vi "PassObserverTactic.vi"(1 "Game in":refnum<class "Game.lvclass">, 8 "error in (no error)":errorcluster, 9 "first call":bool, 10 "Robot":refnum<class "Robot.lvclass">, 11 "PassObserverTactic in":refnum<class "PassObserverTactic.lvclass">) -> (0 "error out":errorcluster, 2 "Robot":refnum<class "Robot.lvclass">, 3 "PassObserverTactic out":refnum<class "PassObserverTactic.lvclass">)   [LabVIEW 2023, in "PassObserverTactic.lvclass"]
uses:
  PassObserverTactic.lvclass
  Robot_class/Robot.lvclass
  Game_class/Game.lvclass
  Utilities_class/Utilities.lvclass
  Robot_class/tactics.ctl
  Tactic_class/Tactic.lvclass/Tactic.ctl
  Skillbook_class/Skillbook.lvclass/Skillbook.ctl
  Game_class/Game.lvclass/Game.ctl
  Robot_class/Robot.lvclass/Robot.ctl
  Game_class/Read Utilities.lvclass.vi
  Game_class/Read BallRef.vi
  Skillbook_class/Read HaltSkill.vi
  Robot_class/Write dest_orientation.vi
  Tactic_class/Read Skillbook.vi
  Robot_class/Write tactic.vi
  Skillbook_class/Skillbook.lvclass
  PassObserverSkill_class/PassObserverSkill.lvclass
  Ball_class/Ball.lvclass
  HaltSkill_class/HaltSkill.lvclass
panel:
  out "x .or. y?":bool
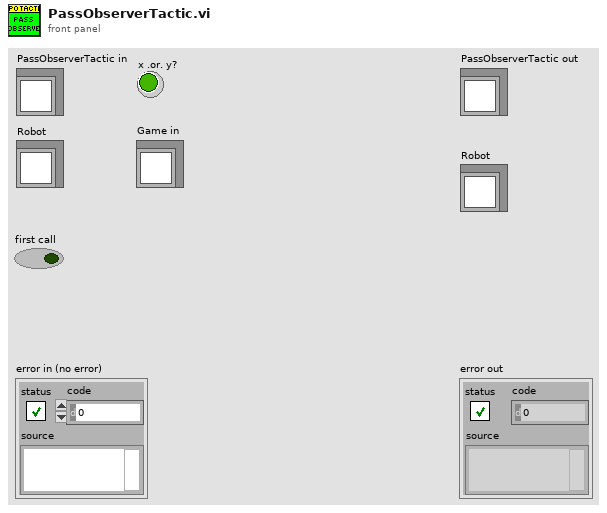
[diagram p1: front panel]
types:
  T1 = typedef "tactics.ctl" = enum16{"ReceivePassInFuturePoint", "Roller", "PrepareRollToPassRollerGoTo", "PrepareRollToPassReceiverGoTo", "WaitRoll", "PositionToRoll", "PenaltyAttacker", "PassObserver", "PenaltyDefense", "TableReceiverTactic", "Test", "DefendGoal", "Marker", "FollowAttacker", "DefendArea", "Shoot", "AttackerAimGoal", "AttackerBallOutOfField", "AttackerBlock", "AttackerStop", "Duelist", "Halt", "ZigZag", "GoTo", "Timeout", "KickToPassReceiver", "PositionToReceivePass", "DefendAreaVSS", "DefendGoalVSS", "KickVSS", "AttackVSS", "DispBallVSS", "PenaltyAttackVSS", "WaitPass"}
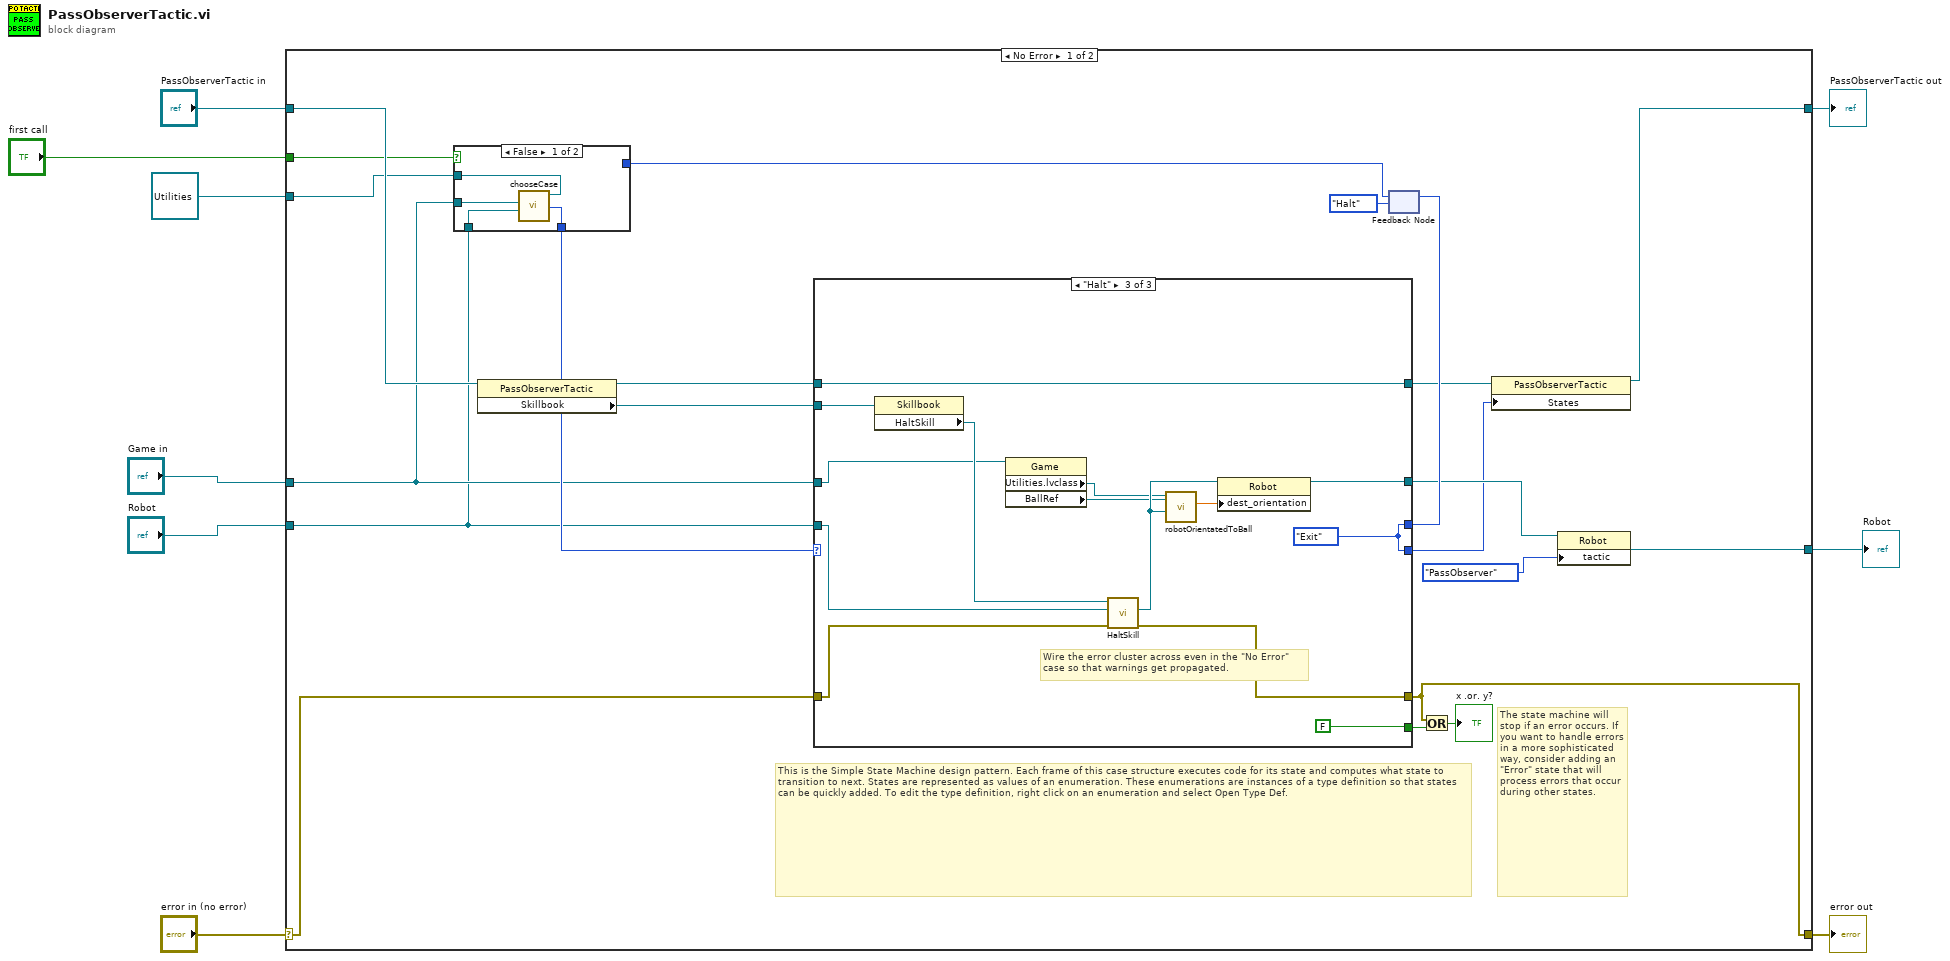
[diagram p0: block diagram]
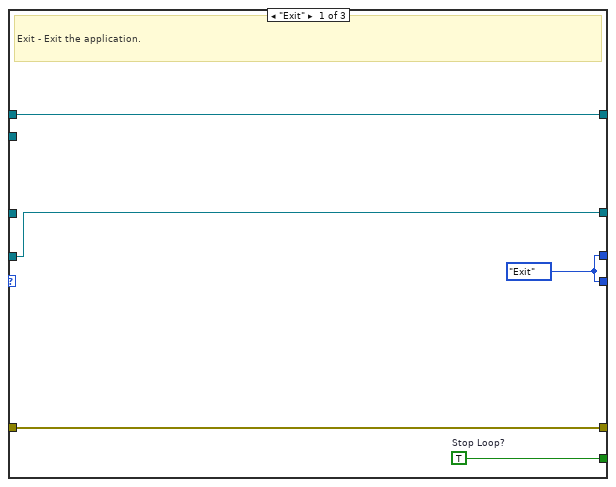
[diagram p2: hidden frame]
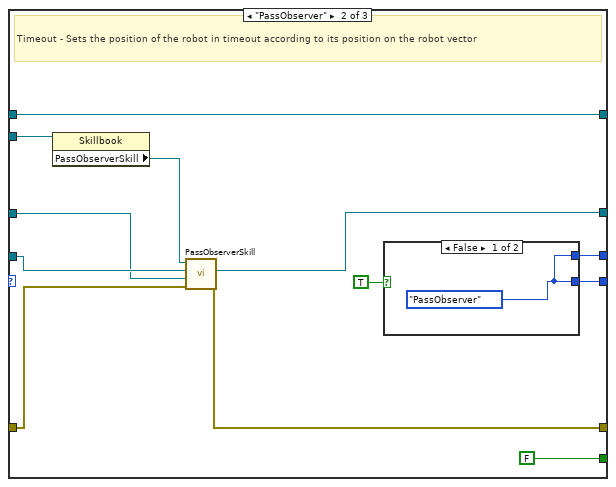
[diagram p3: hidden frame]
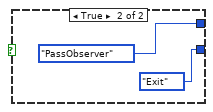
[diagram p4: hidden frame]
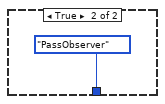
[diagram p5: hidden frame]
diagram:
  n1 = case shown="No Error" "error in (no error)" {
    selector: "error in (no error)" -> [w22 w72]
    tunnel: [w21 w72] -> w8
    tunnel: [w14 w71] -> w6
    tunnel: "PassObserverTactic in" -> [w19 w71]
    tunnel: "Robot" -> [w10 w70]
    tunnel: [w20 w70] -> w4
    tunnel: "first call" -> [w17 _]
    tunnel: "Game in" -> [w11 _]
    tunnel: refnum<class "Utilities.lvclass"> refnum ("Utilities in") -> [w12 _]
    frame No Error {
      # "The state machine will stop if an error occurs. If you want to handle errors in a more sophisticated way, consider adding an \"Error\" state that will process errors that occur during other states."
      # "This is the Simple State Machine design pattern. Each frame of this case structure executes code for its state and computes what state to transition to next. States are represented as values of an enumeration. These enumerations are instances of a type definition so that states can be quickly added. To edit the type definition, right click on an enumeration and select Open Type Def."
      # "Wire the error cluster across even in the \"No Error\"\ncase so that warnings get propagated."
      n2 = property class="PassObserverTactic"(reference=w19) -> (reference out=w27:refnum<class "PassObserverTactic.lvclass">, "Skillbook"=w28:refnum<class "Skillbook.lvclass">)  [unwired: 1 in, 1 out]
      n3 = feedback #1(enum16{"PassObserver", "Halt", "Exit"}."Halt" ("States")) -> (w25:enum16{"PassObserver", "Halt", "Exit"})
      n4 = case shown="False" w17 {
        tunnel: [w68 enum16{"PassObserver", "Halt", "Exit"}."PassObserver" ("States")] -> w16
        tunnel: w25 -> [_ _]
        tunnel: w12 -> [w67 _]
        tunnel: w11 -> [w66 _]
        tunnel: w10 -> [w65 _]
        frame False {
          n5 = call "chooseCase.vi"("Robot"=w65, "Game in"=w66, "Utilities in"=w67) -> ("States"=w68:enum16{"PassObserver", "Halt", "Exit"})  [unwired: 8 in]
        }
        frame True {
        }
      }
      n6 = case shown="\"Halt\"" w16 {
        tunnel: [w31 w44 w58] -> w13
        tunnel: [w35 FALSE ("Stop Loop?") FALSE ("Stop Loop?")] -> w30
        tunnel: w22 -> [w34 w39 w63]
        tunnel: [w34 w38 w62] -> w21
        tunnel: w28 -> [_ w46 w61]
        tunnel: w10 -> [w33 w40 w59]
        tunnel: [w33 w41 w56] -> w23
        tunnel: [w32 w45 w64] -> w15
        tunnel: w27 -> [w32 w45 w64]
        tunnel: [w31 w43 w58] -> w26
        tunnel: w11 -> [_ w37 w53]
        frame "Exit" {
          w31 = enum16{"PassObserver", "Halt", "Exit"}."Exit" ("States")
          w35 = TRUE  # Stop Loop?
          # "Exit - Exit the application."
        }
        frame "PassObserver" {
          # "Timeout - Sets the position of the robot in timeout according to its position on the robot vector"
          n7 = property class="Skillbook"(reference=w46) -> ("PassObserverSkill"=w42:refnum<class "PassObserverSkill.lvclass">)  [unwired: 1 in, 2 out]
          n8 = call-dynamic "PassObserverSkill.vi"("error in (no error)"=w39, "Game in"=w37, "Robot"=w40, "PassObserverSkill in"=w42) -> ("error out"=w38:errorcluster, "Robot"=w41:refnum<class "Robot.lvclass">)  [unwired: 4 in, 2 out]
          n9 = case shown="False" TRUE {
            tunnel: [w48 enum16{"PassObserver", "Halt", "Exit"}."Exit" ("States")] -> w44
            tunnel: [w48 enum16{"PassObserver", "Halt", "Exit"}."PassObserver" ("States")] -> w43
            frame False {
              w48 = enum16{"PassObserver", "Halt", "Exit"}."PassObserver" ("States")
            }
            frame True {
            }
          }
        }
        frame "Halt" {
          w58 = enum16{"PassObserver", "Halt", "Exit"}."Exit" ("States")
          n10 = property class="Skillbook"(reference=w61) -> ("HaltSkill"=w60:refnum<class "HaltSkill.lvclass">)  [unwired: 1 in, 2 out]
          n11 = property class="Game"(reference=w53) -> ("Utilities.lvclass"=w52:refnum<class "Utilities.lvclass">, "BallRef"=w51:refnum<class "Ball.lvclass">)  [unwired: 1 in, 2 out]
          n12 = call-dynamic "HaltSkill.vi"("error in (no error)"=w63, "Robot"=w59, "HaltSkill in"=w60) -> ("error out"=w62:errorcluster, "Robot out"=w54:refnum<class "Robot.lvclass">)  [unwired: 6 in, 1 out]
          n13 = call "robotOrientatedToBall.vi"("Robot"=w54, "BallRef"=w51, "Utilities in"=w52) -> ("Orientation"=w55:dbl)  [unwired: 6 in, 2 out]
          n14 = property class="Robot"(reference=w54, "dest_orientation"=w55) -> (reference out=w56:refnum<class "Robot.lvclass">)  [unwired: 1 in, 1 out]
        }
      }
      n15 = feedback-in #1(w26) -> ()
      n16 = Or(x=w21, y=w30) -> (x .or. y?=→"x .or. y?":bool)
      n17 = property class="PassObserverTactic"(reference=w15, "States"=w13) -> (reference out=w14:refnum<class "PassObserverTactic.lvclass">)  [unwired: 1 in, 1 out]
      n18 = property class="Robot"(reference=w23, "tactic"=tactics."PassObserver") -> (reference out=w20:refnum<class "Robot.lvclass">)  [unwired: 1 in, 1 out]
    }
    frame Error {
      # "Wire the error cluster across even in the \"No Error\"\ncase so that warnings get propagated."
    }
  }
  "error out" <- w8
  "PassObserverTactic out" <- w6
  "Robot" <- w4
